vi "Write CSV File.vi"(8 "error in":errorcluster, 10 "Data":dbl[][](array[numeric]) format="%0.2f", 11 "File Path":path) -> (0 "error out":errorcluster)   [LabVIEW 2021]
doc: "Writes data to a .csv file."
uses:
  <vilib>/Utility/file.llb/Write Delimited Spreadsheet (DBL).vi
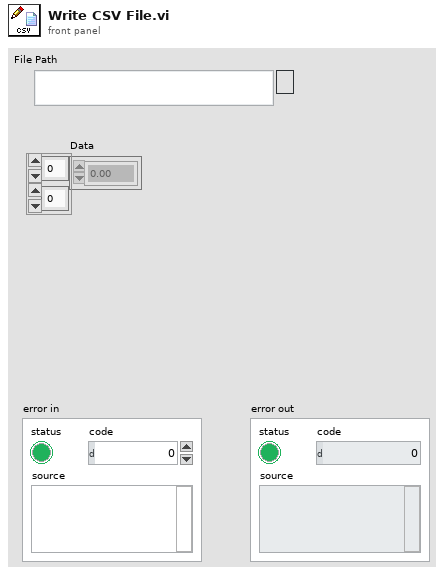
[diagram p1: front panel]
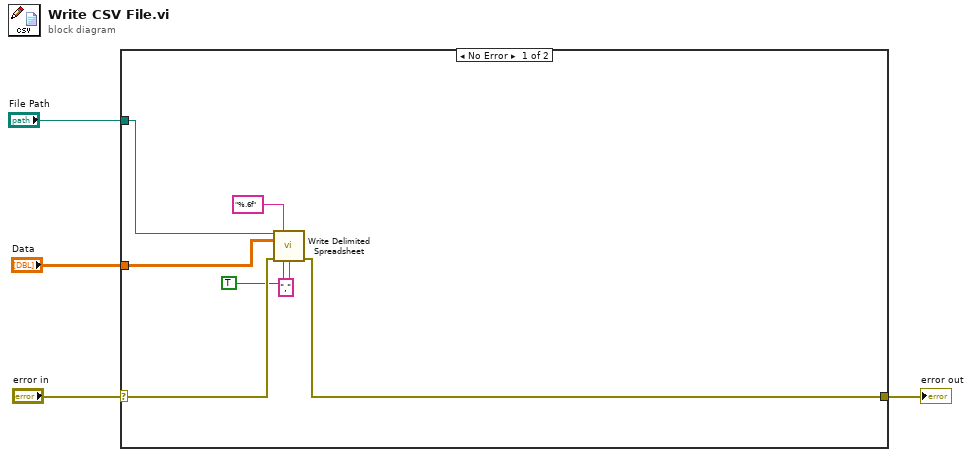
[diagram p0: block diagram]
diagram:
  n1 = case shown="No Error" "error in" {
    selector: "error in" -> [w9 w12]
    tunnel: [w8 w12] -> w3
    tunnel: "File Path" -> [w11 _]
    tunnel: "Data" -> [w10 _]
    frame No Error {
      n2 = call-poly <vilib>:"Write Delimited Spreadsheet.vi"("file path (dialog if empty)"=w11, "format (%.3f)"="%.6f", "2D data"=w10, "error in (no error)"=w9, "transpose? (no:F)"=TRUE, "delimiter (\\t)"="," ("delimiter (\\t)")) -> ("error out"=w8:errorcluster)  [unwired: 8 in, 1 out]
    }
    frame Error {
    }
  }
  "error out" <- w3
